vi "Main.vi"   [LabVIEW 2021]
uses:
  Interface/Interface.lvclass
  Abstract Class/Abstract Class.lvclass
  Concrete Class/Concrete Class.lvclass
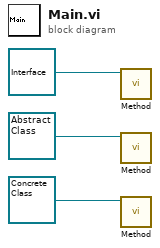
[diagram p0: block diagram]
diagram:
  n1 = call-dynamic "Method.vi"("Interface in"=refnum<class "Interface.lvclass"> refnum ("Interface.lvclass")) -> ()  [unwired: 9 in, 2 out]
  n2 = call-dynamic "Method.vi"("Abstract Class in"=refnum<class "Abstract Class.lvclass"> refnum ("Abstract Class.lvclass")) -> ()  [unwired: 9 in, 2 out]
  n3 = call-dynamic "Method.vi"("Concrete Class in"=refnum<class "Concrete Class.lvclass"> refnum ("Concrete Class.lvclass")) -> ()  [unwired: 9 in, 2 out]
